vi "MuC_Read_SMPL.vi"(3 "error in (no error)":errorcluster, 4 "Tsmpl / us":i32, 5 "VISA resource name":refnum<visa-resource-name>) -> (0 "error out":errorcluster, 1 "Cmd":string, 2 "VISA resource name 2":refnum<visa-resource-name>)   [LabVIEW 2019]
doc: "Send a command to a MicroController telling it to sample data\n\nThe command for SMPL read as understood by the microcontroller is 's<Tsmpl>'\n\nTsmpl is sampling period in units of micro-seconds in the range [5, 15000]\n\nR. Sheehan 25 - 1 - 2021"
uses:
  <vilib>/regexp/Match Regular Expression.xnode
panel:
  out "return count":u32
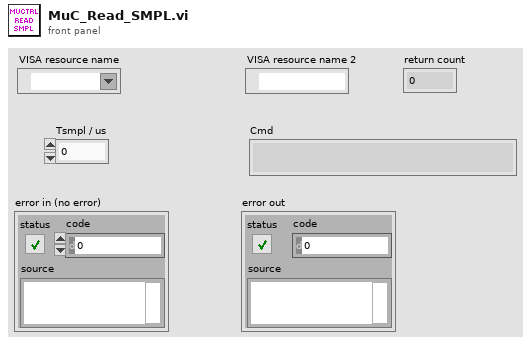
[diagram p1: front panel]
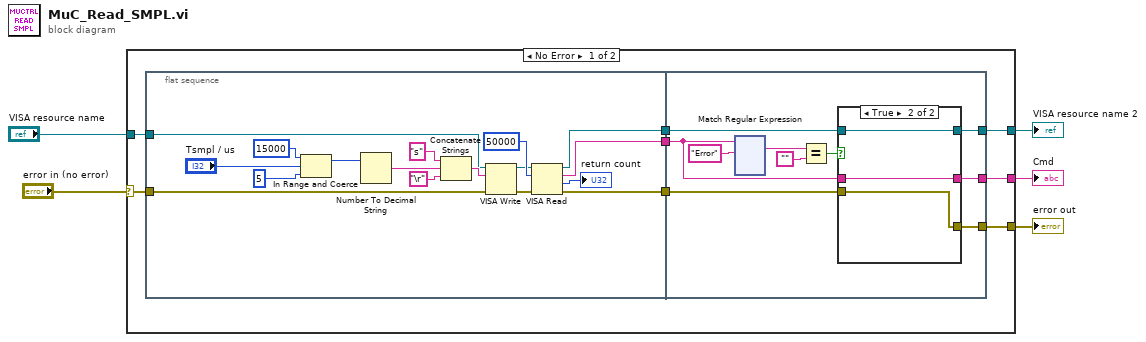
[diagram p0: block diagram]
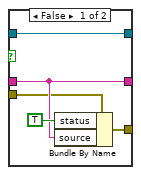
[diagram p2: hidden frame]
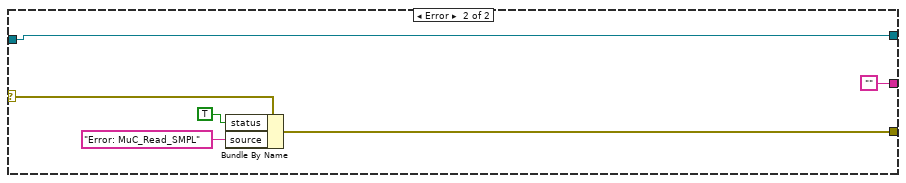
[diagram p3: hidden frame]
diagram:
  n1 = case shown="No Error" "error in (no error)" {
    selector: "error in (no error)" -> [w12 w168]
    tunnel: [w8 w167] -> w4
    tunnel: "VISA resource name" -> [w13 w164]
    tunnel: [w6 w164] -> w2
    tunnel: [w10 ""] -> w1
    frame No Error {
      n2 = flat-sequence {
        tunnel: [w23] -> w11
        tunnel: [w22] -> w9
        tunnel: [w21] -> w7
        tunnel: w13 -> [w25]
        tunnel: w12 -> [w24]
        tunnel: w11 -> [w36]
        tunnel: [w35] -> w10
        tunnel: w9 -> [w34]
        tunnel: [w33] -> w8
        tunnel: w7 -> [w32]
        tunnel: [w31] -> w6
        frame #0 {
          n3 = In Range and Coerce(upper limit=15000, x="Tsmpl / us", lower limit=5) -> (coerced(x)=w18:i32)  [unwired: 1 out]
          n4 = Number To Decimal String(number=w18) -> (decimal integer string=w14:string)  [unwired: 1 in]
          n5 = Concatenate Strings("s" ("string"), w14, "\r") -> (w26:string)
          n6 = VISA Write(VISA resource name=w25, write buffer=w26, error in (no error)=w24) -> (VISA resource name out=w27:refnum<visa-resource-name>, error out=w28:errorcluster)  [unwired: 1 out]
          n7 = VISA Read(VISA resource name=w27, byte count=u32 50000, error in (no error)=w28) -> (VISA resource name out=w21:refnum<visa-resource-name>, read buffer=w23:string, return count=→"return count":u32, error out=w22:errorcluster)
        }
        frame #1 {
          n8 = xnode "Match Regular Expression"("input string"=w36, "regular expression"="Error") -> ("whole match"=w38:string)  [unwired: 4 in, 4 out]
          n9 = Equal?(x=w38, y="") -> (x = y?=w37:bool)
          n10 = case shown="True" w37 {
            tunnel: [w44 w46] -> w33
            tunnel: w36 -> [w43 w47]
            tunnel: [w43 w47] -> w35
            tunnel: w34 -> [w42 w46]
            tunnel: w32 -> [w41 w48]
            tunnel: [w41 w48] -> w31
            frame False {
              n11 = Bundle By Name(cluster=w42, "status"=TRUE, "source"=w43) -> (w44:errorcluster)
            }
            frame True {
            }
          }
        }
      }
    }
    frame Error {
      n12 = Bundle By Name(cluster=w168, "status"=TRUE, "source"="Error: MuC_Read_SMPL") -> (w167:errorcluster)
    }
  }
  "error out" <- w4
  "VISA resource name 2" <- w2
  "Cmd" <- w1
